vi "barcode serial no incriment.vi"(11 "Serial No":string="0166") -> (0 "serial no incriment":string="0166", 2 "go in printer":string="0166")   [LabVIEW 2015]
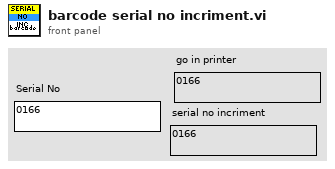
[diagram p1: front panel]
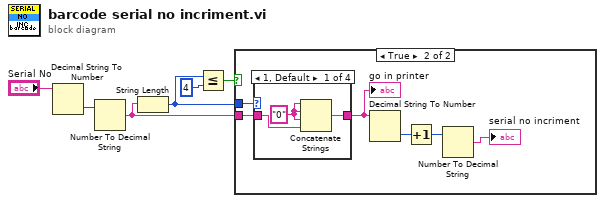
[diagram p0: block diagram]
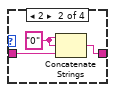
[diagram p3: hidden frame]
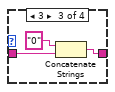
[diagram p4: hidden frame]
diagram:
  n1 = Decimal String To Number(string="Serial No") -> (number=w5:i32)  [unwired: 2 in, 1 out]
  n2 = Number To Decimal String(number=w5) -> (decimal integer string=w4:string)  [unwired: 1 in]
  n3 = String Length(string=w4) -> (length=w2:i32)
  n4 = Less Or Equal?(x=w2, y=4) -> (x <= y?=w3:bool)
  n5 = case shown="True" w3 {
    tunnel: w2 -> [_ w12]
    tunnel: w4 -> [_ w8]
    frame False {
    }
    frame True {
      n6 = case shown="1, Default" w12 {
        tunnel: w8 -> [w14 w16 w20 w22]
        tunnel: [w13 w17 w19 w22] -> w10
        frame 1, Default {
          w15 = "0" ("string")
          n7 = Concatenate Strings(w15, w15, w15, w14) -> (w13:string)
        }
        frame 2 {
          w18 = "0" ("string")
          n8 = Concatenate Strings(w18, w18, w16) -> (w17:string)
        }
        frame 3 {
          n9 = Concatenate Strings("0" ("string"), w20) -> (w19:string)
        }
        frame 4 {
        }
      }
      "go in printer" <- w10
      n10 = Decimal String To Number(string=w10) -> (number=w11:i32)  [unwired: 2 in, 1 out]
      n11 = Increment(x=w11) -> (x+1=w9:i32)
      n12 = Number To Decimal String(number=w9) -> (decimal integer string=→"serial no incriment":string)  [unwired: 1 in]
    }
  }
